vi "PS2000.vi"() -> ()   [LabVIEW 2016]
uses:
  <vilib>/measure/mascope.llb/Amplitude and Levels 1 chan.vi
  <vilib>/measure/matone.llb/Extract Single Tone Information 1 Chan.vi
  <vilib>/measure/mascope.llb/Pulse Measurements 1 chan.vi
  PS2000.dll
  <vilib>/measure/NI_MAPro.lvlib
panel:
  out "Phase":dbl
  out "Low level":dbl
  out "High level":dbl
  out "Amplitude":dbl
  out "Phase":dbl
  out "Behind":bool
  out "Advance":bool
  out "Low level":dbl
  out "High level":dbl
  out "Amplitude":dbl
  out "Phase difference":dbl
  out "Duty cycle":dbl
  out "Period":dbl
  out "Duty cycle":dbl
  out "Period":dbl
  in  "Voltage Range":dbl(knob) min=0.0 max=20.0 step=0.001 scale=0.0..20.0
  in  "Time":dbl(knob) min=0.0 max=1.0 step=0.0001 scale=0.0..1.0
  in  "stop 2":bool
  in  "Sweeps":u32
  in  "Sweep Type":u16(ring) items=["Up", "Down", "Up/Down", "Down/Up"]
  in  "Dwell Time":sgl
  in  "Increment":sgl
  in  "Stop Frequency":sgl=1000.0
  in  "Start Frequency":sgl=1000.0
  in  "Waveform Type":u16(ring) items=["Sine", "Square", "Triangle", "Rampup", "Rampdown"]
  in  "Peak to Peak":u32=1000000
  in  "Offset Voltage":i32
  in  "Source":i16(ring)=5 items=["Ch A", "Ch B", "Ch C", "Ch D", "Ext", "None"]
  in  "Voltage mV":i16=1400 min=0 max=20000 step=1
  out "Handle":u16
  out "Max number of samples you can use":i32=15871
  in  "Range":i16(ring)=5 items=["20V"=10, "10V"=9, "5V"=8, "2V"=7, "1V"=6, "500mV"=5, "200mV"=4, "100mV"=3, "50mV"=2]
  in  "Range":i16(ring)=8 items=["20V"=10, "10V"=9, "5V"=8, "2V"=7, "1V"=6, "500mV"=5, "200mV"=4, "100mV"=3, "50mV"=2]
  out "?":waveform(dbl)[](graph)=[{"t0"=timestamp(3286802554.3350306 s since 1904-01-01), "dt"=5.024e-05, "Y"=array[1256 elements]}, {"t0"=timestamp(3286802554.3350306 s since 1904-01-01), "dt"=5.024e-05, "Y"=array[1256 elements]}, {"t0"=timestamp(3286802554.3350306 s since 1904-01-01), "dt"=5.024e-05, "Y"=array[1256 elements]}, {"t0"=timestamp(3286802554.3350306 s since 1904-01-01), "dt"=5.024e-05, "Y"=array[1256 elements]}]
  in  "Enabled":bool
  in  "Enabled":bool=TRUE
  in  "DC":i16(ring) items=["AC", "DC"]
  in  "DC":i16(ring)=1 items=["AC", "DC"]
  in  "No. of samples":i32=1256 min=0
  in  "Timebase":i16=3 min=0 max=14 step=1
  in  "Auto Trigger ms":i16 min=0 max=5000 step=100
  in  "Delay":i16 min=-100 max=100 step=1
  in  "Direction":i16(ring) items=["Rising", "Falling"]
  in  "stop":bool
  # "Computer Oscilloscope"
  # "(Edition: Automatic Performance Test For Encoders )"
  # "Channel A"
  # "Channel B"
  # "Timebase"
  # "Trigger"
  # "AWG"
  # "Channel A"
  # "Channel B"
  # "Special function"
  # "V.2016.9.13.1"
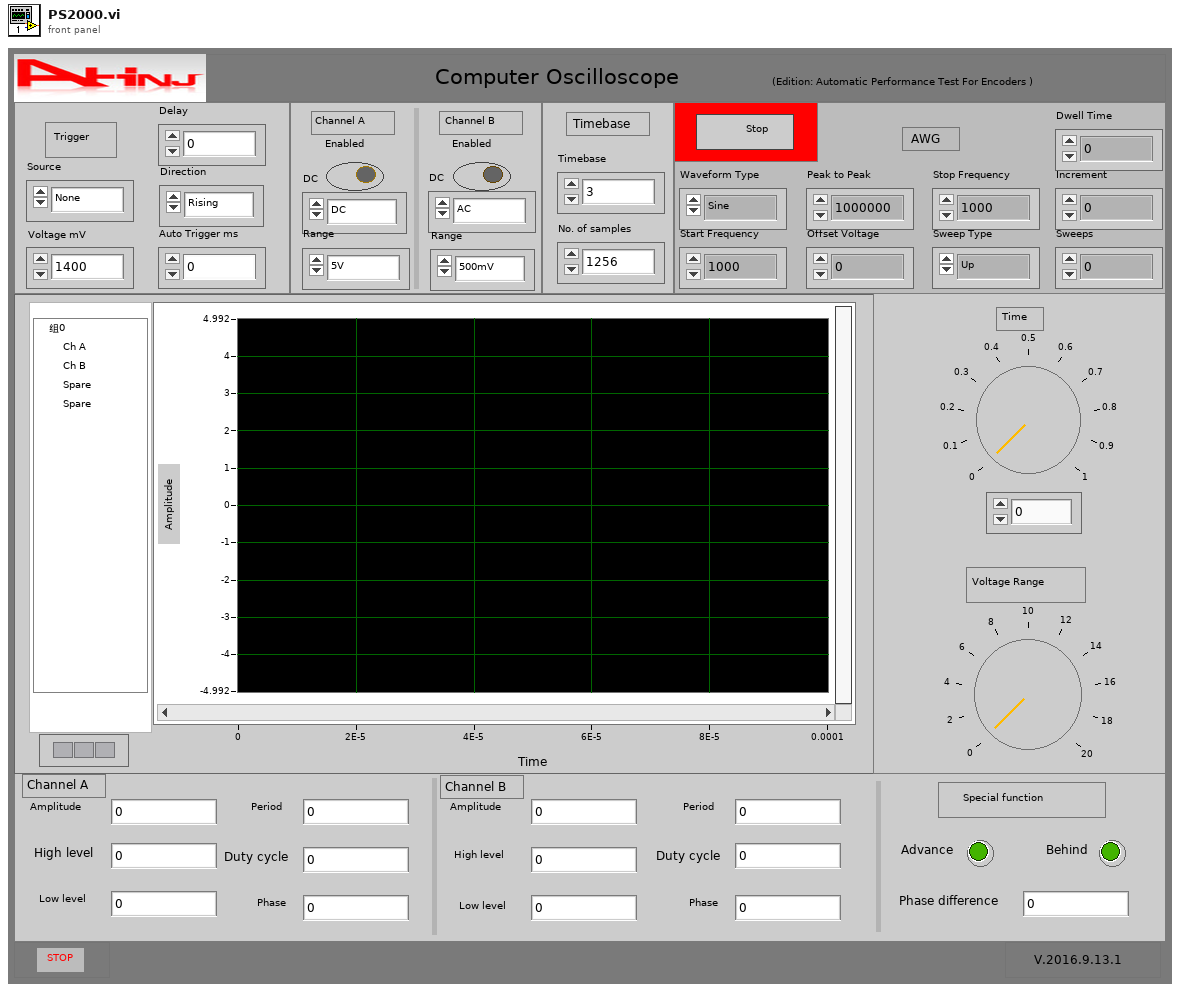
[diagram p1: front panel]
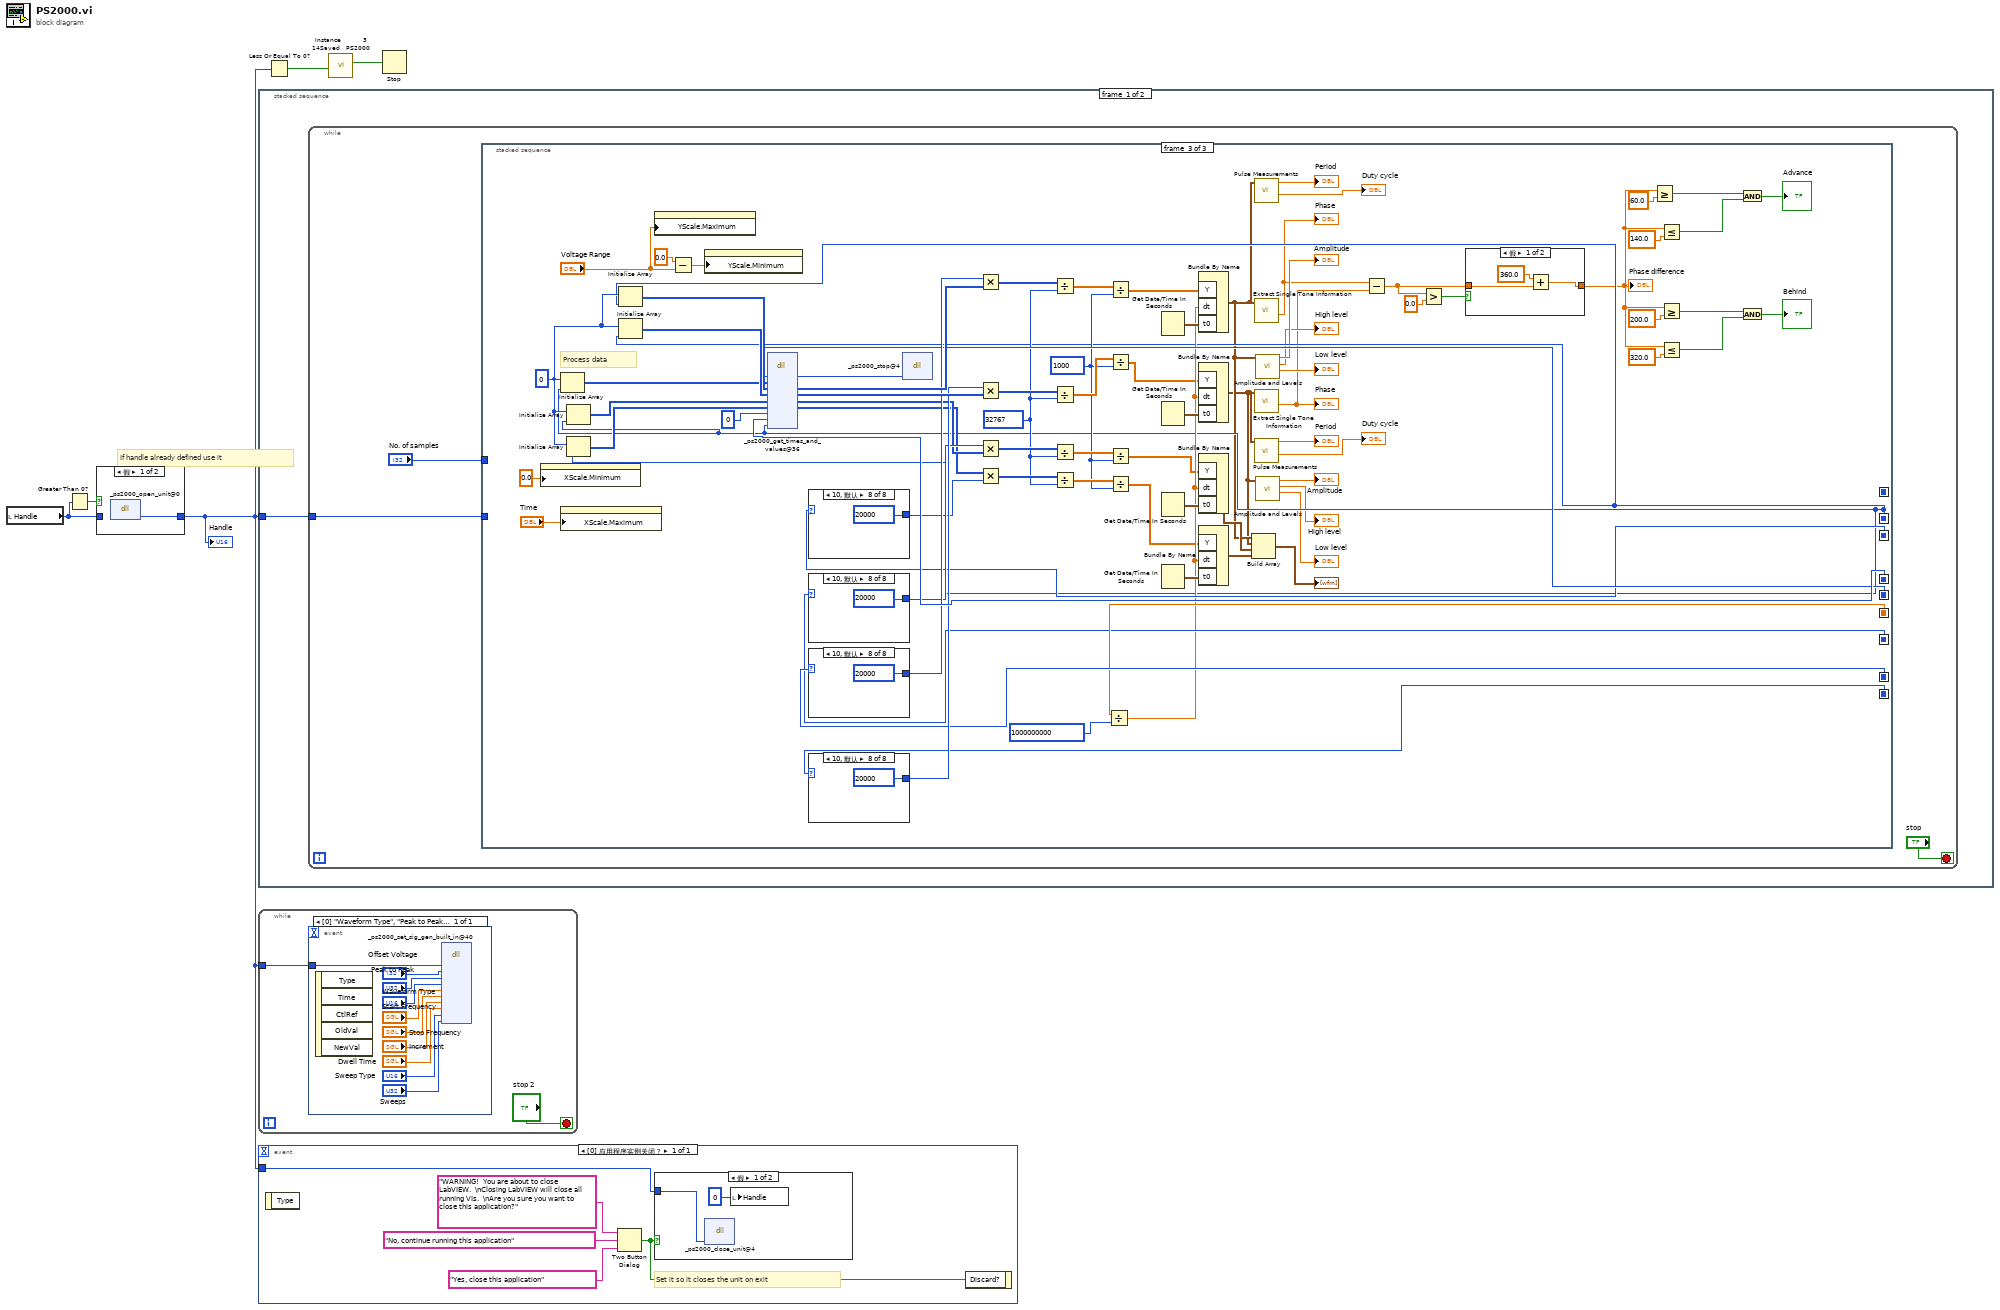
[diagram p0: block diagram]
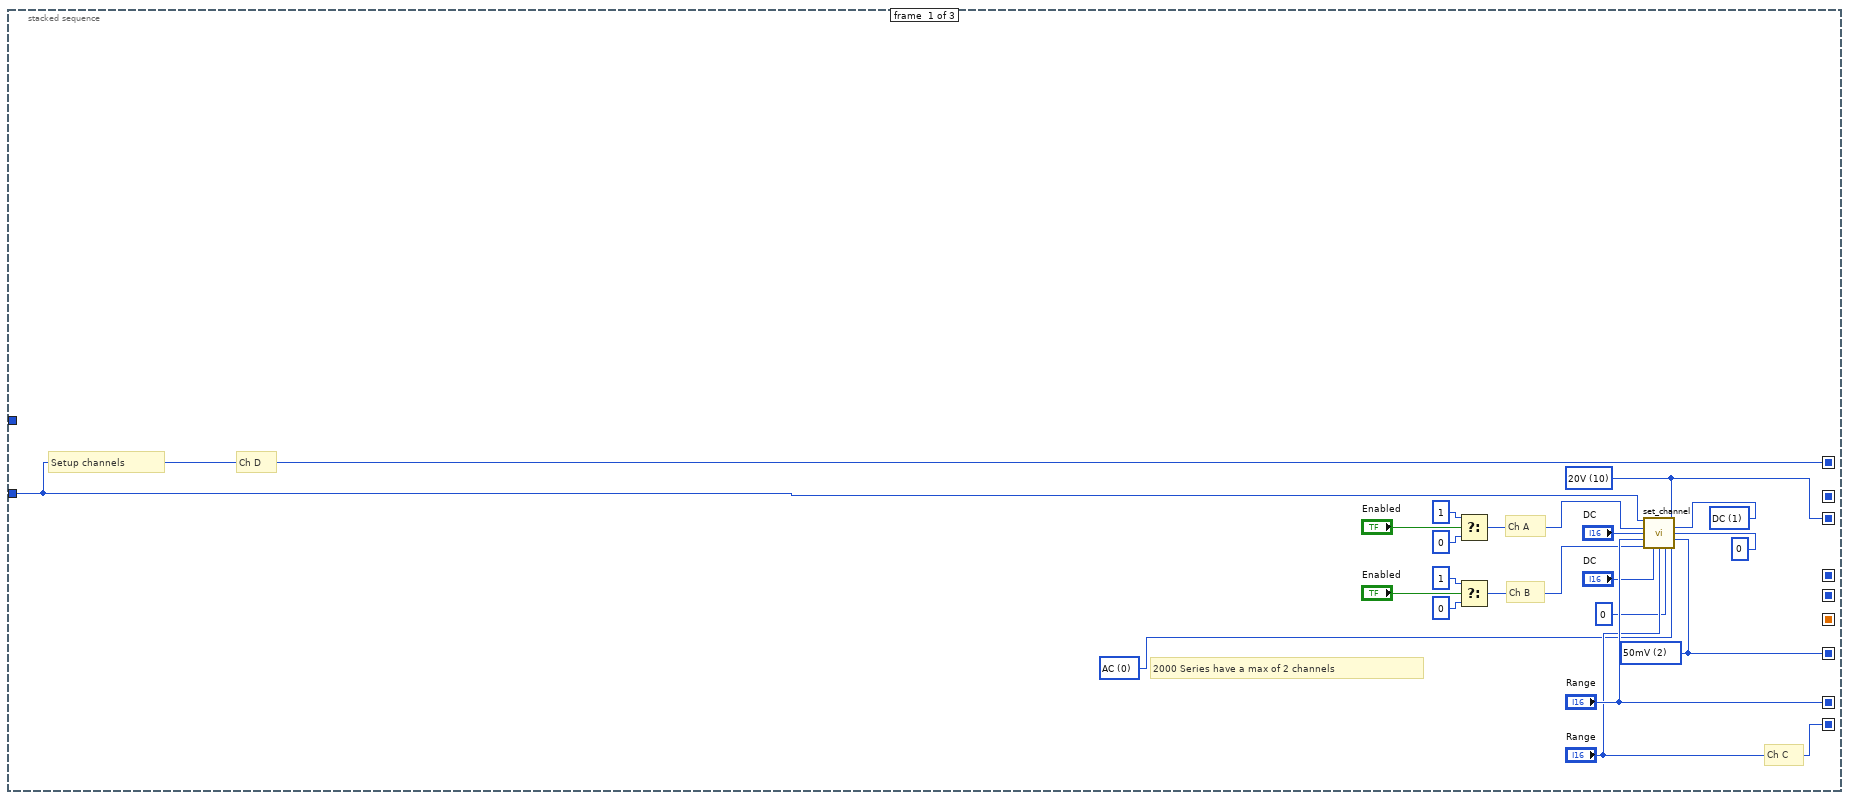
[diagram p3: hidden frame]
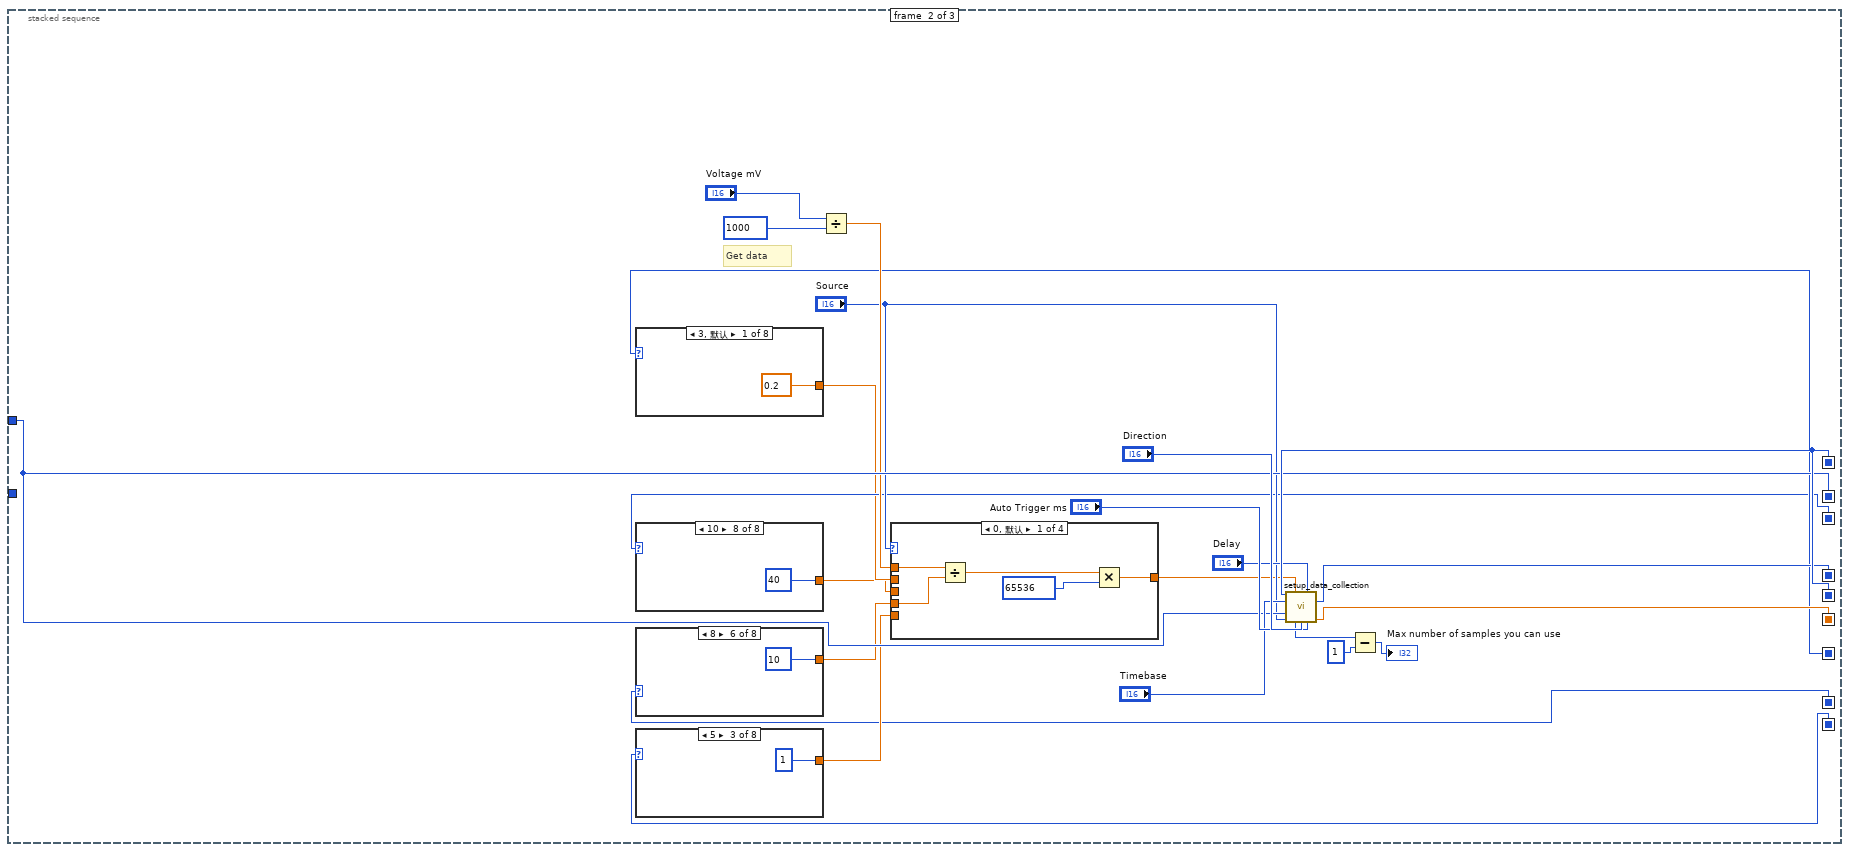
[diagram p4: hidden frame]
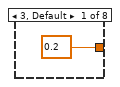
[diagram p5: hidden frame]
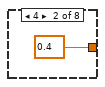
[diagram p6: hidden frame]
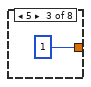
[diagram p7: hidden frame]
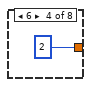
[diagram p8: hidden frame]
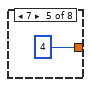
[diagram p9: hidden frame]
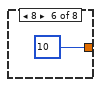
[diagram p10: hidden frame]
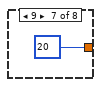
[diagram p11: hidden frame]
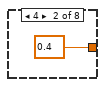
[diagram p12: hidden frame]
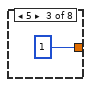
[diagram p13: hidden frame]
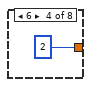
[diagram p14: hidden frame]
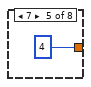
[diagram p15: hidden frame]
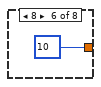
[diagram p16: hidden frame]
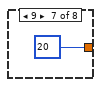
[diagram p17: hidden frame]
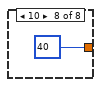
[diagram p18: hidden frame]
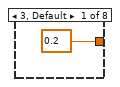
[diagram p19: hidden frame]
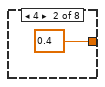
[diagram p20: hidden frame]
diagram:
  # "If handle already defined use it"
  n1 = local read "Handle"() -> (w4:u16)
  n2 = Greater Than 0?(x=w4) -> (x > 0?=w5:bool)
  n3 = case shown="假" w5 {
    tunnel: [w6 w7] -> w1
    tunnel: w4 -> [_ w7]
    frame False {
      n4 = dll-call lib="PS2000.dll" fn="_ps2000_open_unit@0" label="OpenUnit"() -> ("Handle"=w6:i16)  [unwired: 3 in, 2 out]
    }
    frame True {
    }
  }
  "Handle" <- w1
  n5 = stacked-sequence {
    tunnel: w1 -> [w8 _]
    frame #0 {
      n6 = while {
        tunnel: w8 -> [w10]
        stop <- "stop" stop-if-true
        n7 = stacked-sequence {
          seq-local: [w24 _ _] -> [_ w51 _]
          seq-local: [_ w51 _] -> [_ _ w168]
          seq-local: [_ w49 _] -> [_ _ w144]
          seq-local: [_ w50 _] -> [_ _ w182]
          seq-local: ["Range" _ _] -> [_ w36 w169]
          seq-local: ["Range" _ _] -> [_ w37 w170]
          seq-local: [_ w48 _] -> [_ _ w166]
          seq-local: [w15 _ _] -> [_ w34 w155]
          seq-local: [w14 _ _] -> [_ w33 w154]
          tunnel: w10 -> [w24 _ _]
          tunnel: "No. of samples" -> [_ w49 _]
          frame #0 {
            w16 = i16 1 items=["AC", "DC"] ("DC")
            w14 = i16 10 items=["20V"=10, "10V"=9, "5V"=8, "2V"=7, "1V"=6, "500mV"=5, "200mV"=4, "100mV"=3, "50mV"=2] ("Range")
            w17 = i16 0 items=["AC", "DC"] ("DC")
            w15 = i16 2 items=["20V"=10, "10V"=9, "5V"=8, "2V"=7, "1V"=6, "500mV"=5, "200mV"=4, "100mV"=3, "50mV"=2] ("Range")
            # "2000 Series have a max of 2 channels"
            # "Ch C"
            # "Ch D"
            # "Ch B"
            # "Ch A"
            # "Setup channels"
            n8 = Select(t=1, s="Enabled", f=0) -> (s? t:f=w23:i32)
            n9 = Select(t=1, s="Enabled", f=0) -> (s? t:f=w20:i32)
            n10 = call "set_channel.vi"("Handle"=w24, "Channel D range"=w14, "Channel A enabled"=w23, "Channel D dc"=w16, "Channel A dc"="DC", "Channel D enabled"=0, "Channel A range"="Range", "Channel C range"=w15, "Channel B enabled"=w20, "Channel B dc"="DC", "Channel B range"="Range", "Channel C enabled"=0, "Channel C dc"=w17) -> ()  [unwired: 3 in]
          }
          frame #1 {
            # "Get data"
            n11 = case shown="3, 默认" w34 {
              tunnel: [0.2 0.4 1 2 4 10 20 40] -> w32
              frame 3, Default {
              }
              frame 4 {
              }
              frame 5 {
              }
              frame 6 {
              }
              frame 7 {
              }
              frame 8 {
              }
              frame 9 {
              }
              frame 10 {
              }
            }
            n12 = case shown="10" w33 {
              tunnel: [0.2 0.4 1 2 4 10 20 40] -> w31
              frame 3, Default {
              }
              frame 4 {
              }
              frame 5 {
              }
              frame 6 {
              }
              frame 7 {
              }
              frame 8 {
              }
              frame 9 {
              }
              frame 10 {
              }
            }
            n13 = case shown="8" w36 {
              tunnel: [0.2 0.4 1 2 4 10 20 40] -> w40
              frame 3, Default {
              }
              frame 4 {
              }
              frame 5 {
              }
              frame 6 {
              }
              frame 7 {
              }
              frame 8 {
              }
              frame 9 {
              }
              frame 10 {
              }
            }
            n14 = case shown="5" w37 {
              tunnel: [0.2 0.4 1 2 4 10 20 40] -> w39
              frame 3, Default {
              }
              frame 4 {
              }
              frame 5 {
              }
              frame 6 {
              }
              frame 7 {
              }
              frame 8 {
              }
              frame 9 {
              }
              frame 10 {
              }
            }
            n15 = Divide(x="Voltage mV", y=1000) -> (x/y=w41:dbl)
            n16 = case shown="0, 默认" "Source" {
              tunnel: w40 -> [w90 _ _ _]
              tunnel: w39 -> [_ w92 _ _]
              tunnel: w41 -> [w91 w93 w98 w103]
              tunnel: [w87 w94 w99 w104] -> w35
              tunnel: w32 -> [_ _ w97 _]
              tunnel: w31 -> [_ _ _ w102]
              frame 0, Default {
                n17 = Divide(x=w91, y=w90) -> (x/y=w89:dbl)
                n18 = Multiply(x=w89, y=65536) -> (x*y=w87:dbl)
              }
              frame 1 {
                n19 = Divide(x=w93, y=w92) -> (x/y=w96:dbl)
                n20 = Multiply(x=w96, y=65536) -> (x*y=w94:dbl)
              }
              frame 2 {
                n21 = Divide(x=w98, y=w97) -> (x/y=w101:dbl)
                n22 = Multiply(x=w101, y=65536) -> (x*y=w99:dbl)
              }
              frame 3 {
                n23 = Divide(x=w103, y=w102) -> (x/y=w106:dbl)
                n24 = Multiply(x=w106, y=65536) -> (x*y=w104:dbl)
              }
            }
            n25 = call "setup_data_collection.vi"("Handle"=w51, "Threshold"=w35, "Delay"="Delay", "Timebase"="Timebase", "No of samples"=w49, "Source"="Source", "Direction"="Direction", "Auto Trigger ms"="Auto Trigger ms") -> ("time units"=w50:i16, "Max Samples"=w45:i32, "time_interval_ns"=w48:dbl)  [unwired: 3 in, 2 out]
            n26 = Subtract(x=w45, y=1) -> (x-y=→"Max number of samples you can use":i32)
          }
          frame #2 {
            w158 = 1000
            w159 = 32767
            w145 = 0
            # "Process data"
            n27 = property class="MixedGraph (严格)"("XScale.Minimum"=0.0) -> ()  [unwired: 2 in, 2 out]
            n28 = Initialize Array(w145, w144) -> (w142:i32[])
            n29 = property class="MixedGraph (严格)"("XScale.Maximum"="Time") -> ()  [unwired: 2 in, 2 out]
            n30 = Initialize Array(w145, w144) -> (w184:i32[])
            n31 = Initialize Array(w145, w144) -> (w183:i32[])
            n32 = Initialize Array(w145, w144) -> (w186:i32[])
            n33 = Initialize Array(w145, w144) -> (w185:i32[])
            n34 = property class="MixedGraph (严格)"("YScale.Maximum"="Voltage Range") -> ()  [unwired: 2 in, 2 out]
            n35 = Subtract(x=0.0, y="Voltage Range") -> (x-y=w139:dbl)
            n36 = property class="MixedGraph (严格)"("YScale.Minimum"=w139) -> ()  [unwired: 2 in, 2 out]
            n37 = dll-call lib="PS2000.dll" fn="_ps2000_get_times_and_values@36" label="GetTimes&Values"("handle"=w168, "times"=w142, "bufferA"=w186, "bufferB"=w185, "bufferC"=w184, "bufferD"=w183, "overflow"=0, "times_units"=w182, "numValues"=w144) -> ("handle"=w178:i16, "bufferA"=w179:i16[], "bufferB"=w173:i16[], "bufferC"=w157:i16[], "bufferD"=w156:i16[])  [unwired: 8 in, 2 out]
            n38 = case shown="10, 默认" w154 {
              tunnel: [100 200 500 1000 2000 5000 10000 20000] -> w160
              frame 3 {
              }
              frame 4 {
              }
              frame 5 {
              }
              frame 6 {
              }
              frame 7 {
              }
              frame 8 {
              }
              frame 9 {
              }
              frame 10, Default {
              }
            }
            n39 = case shown="10, 默认" w155 {
              tunnel: [100 200 500 1000 2000 5000 10000 20000] -> w161
              frame 3 {
              }
              frame 4 {
              }
              frame 5 {
              }
              frame 6 {
              }
              frame 7 {
              }
              frame 8 {
              }
              frame 9 {
              }
              frame 10, Default {
              }
            }
            n40 = case shown="10, 默认" w169 {
              tunnel: [100 200 500 1000 2000 5000 10000 20000] -> w171
              frame 3 {
              }
              frame 4 {
              }
              frame 5 {
              }
              frame 6 {
              }
              frame 7 {
              }
              frame 8 {
              }
              frame 9 {
              }
              frame 10, Default {
              }
            }
            n41 = case shown="10, 默认" w170 {
              tunnel: [100 200 500 1000 2000 5000 10000 20000] -> w172
              frame 3 {
              }
              frame 4 {
              }
              frame 5 {
              }
              frame 6 {
              }
              frame 7 {
              }
              frame 8 {
              }
              frame 9 {
              }
              frame 10, Default {
              }
            }
            n42 = dll-call lib="PS2000.dll" fn="_ps2000_stop@4" label="Stop"("handle"=w178) -> ()  [unwired: 5 in, 2 out]
            n43 = Multiply(x=w171, y=w179) -> (x*y=w181:i32[])
            n44 = Multiply(x=w172, y=w173) -> (x*y=w176:i32[])
            n45 = Multiply(x=w161, y=w157) -> (x*y=w165:i32[])
            n46 = Multiply(x=w156, y=w160) -> (x*y=w163:i32[])
            n47 = Divide(x=w181, y=w159) -> (x/y=w180:dbl[])
            n48 = Divide(x=w176, y=w159) -> (x/y=w175:dbl[])
            n49 = Divide(x=w165, y=w159) -> (x/y=w164:dbl[])
            n50 = Divide(x=w163, y=w159) -> (x/y=w162:dbl[])
            n51 = Divide(x=w166, y=1000000000) -> (x/y=w151:dbl)
            n52 = Divide(x=w180, y=w158) -> (x/y=w125:dbl[])
            n53 = Divide(x=w175, y=w158) -> (x/y=w136:dbl[])
            n54 = Divide(x=w164, y=w158) -> (x/y=w147:dbl[])
            n55 = Divide(x=w162, y=w158) -> (x/y=w146:dbl[])
            n56 = Get Date/Time In Seconds() -> (seconds since 1Jan1904=w177:timestamp)
            n57 = Get Date/Time In Seconds() -> (seconds since 1Jan1904=w174:timestamp)
            n58 = Get Date/Time In Seconds() -> (seconds since 1Jan1904=w153:timestamp)
            n59 = Get Date/Time In Seconds() -> (seconds since 1Jan1904=w152:timestamp)
            n60 = Bundle By Name("Y"=w125, "dt"=w151, "t0"=w177) -> (w113:waveform(dbl))  [unwired: 1 in]
            n61 = Bundle By Name("Y"=w136, "dt"=w151, "t0"=w174) -> (w111:waveform(dbl))  [unwired: 1 in]
            n62 = Bundle By Name("Y"=w147, "dt"=w151, "t0"=w153) -> (w149:waveform(dbl))  [unwired: 1 in]
            n63 = Bundle By Name("Y"=w146, "dt"=w151, "t0"=w152) -> (w150:waveform(dbl))  [unwired: 1 in]
            n64 = Build Array(w113, w111, w149, w150) -> (→"?":waveform(dbl)[])
            n65 = call-poly <vilib>:"Pulse Measurements.vi"("signal in"=w113) -> ("duty cycle"=→"Duty cycle":dbl, "period"=→"Period":dbl)  [unwired: 6 in, 3 out]
            n66 = call-poly <vilib>:"Extract Single Tone Information.vi"("time signal in"=w113) -> ("detected phase (deg)"=w112:dbl)  [unwired: 5 in, 5 out]
            "Phase" <- w112
            n67 = call-poly <vilib>:"Extract Single Tone Information.vi"("time signal in"=w111) -> ("detected phase (deg)"=w107:dbl)  [unwired: 5 in, 5 out]
            "Phase" <- w107
            n68 = call-poly <vilib>:"Pulse Measurements.vi"("signal in"=w111) -> ("duty cycle"=→"Duty cycle":dbl, "period"=→"Period":dbl)  [unwired: 6 in, 3 out]
            n69 = call-poly <vilib>:"Amplitude and Levels.vi"("signal in"=w113) -> ("low state level"=→"Low level":dbl, "high state level"=→"High level":dbl, "amplitude"=→"Amplitude":dbl)  [unwired: 7 in, 1 out]
            n70 = call-poly <vilib>:"Amplitude and Levels.vi"("signal in"=w111) -> ("low state level"=→"Low level":dbl, "high state level"=→"High level":dbl, "amplitude"=→"Amplitude":dbl)  [unwired: 7 in, 1 out]
            n71 = Subtract(x=w112, y=w107) -> (x-y=w129:dbl)
            n72 = Greater?(x=w129, y=0.0) -> (0:w130:bool)
            n73 = case shown="假" w130 {
              tunnel: w129 -> [w189 w190]
              tunnel: [w187 w190] -> w116
              frame False {
                n74 = Add(x=360.0, y=w189) -> (x+y=w187:dbl)
              }
              frame True {
              }
            }
            "Phase difference" <- w116
            n75 = Greater Or Equal?(x=w116, y=60.0) -> (x >= y?=w121:bool)
            n76 = Less Or Equal?(x=w116, y=140.0) -> (x <= y?=w122:bool)
            n77 = Greater Or Equal?(x=w116, y=200.0) -> (x >= y?=w118:bool)
            n78 = Less Or Equal?(x=w116, y=320.0) -> (x <= y?=w119:bool)
            n79 = And(x=w121, y=w122) -> (x .and. y?=→"Advance":bool)
            n80 = And(x=w118, y=w119) -> (x .and. y?=→"Behind":bool)
          }
        }
      }
    }
    frame #1 {
      n81 = Stop(stop? (T)=TRUE) -> ()
    }
  }
  n82 = while {
    tunnel: w1 -> [w225]
    stop <- "stop 2" stop-if-true
    n83 = event shown="[0] \"Waveform Type\", \"Peak to Peak\", \"Offset Voltage\", \"Stop Frequency\", \"Increment\", \"Dwell Time\", \"Sweep Type\", \"Sweeps\": 值改变" {
      selector: _ -> [_]
      dyn-events: _ -> [_]
      timeout: _ -> [_]
      tunnel: w225 -> [w226]
      event "Waveform Type", "Peak to Peak", "Offset Voltage", "Stop Frequency", "Increment", "Dwell Time", "Sweep Type", "Sweeps": Value Change {
        n84 = event-data() -> ()  [unwired: 1 in, 5 out]
        n85 = dll-call lib="PS2000.dll" fn="_ps2000_set_sig_gen_built_in@40"("handle"=w226, "offsetvoltage"="Offset Voltage", "pktopk"="Peak to Peak", "wavetype"="Waveform Type", "startfrequency"="Start Frequency", "stopfrequency"="Stop Frequency", "increment"="Increment", "dwelltime"="Dwell Time", "sweeptype"="Sweep Type", "sweeps"="Sweeps") -> ()  [unwired: 14 in, 2 out]
      }
    }
  }
  n86 = event shown="[0] 应用程序实例关闭？" {
    selector: _ -> [_]
    dyn-events: _ -> [_]
    timeout: _ -> [_]
    tunnel: w1 -> [w236]
    event Application Instance Close? {
      # "Set it so it closes the unit on exit"
      n87 = event-data() -> ()  [unwired: 1 in, 1 out]
      n88 = Two Button Dialog(message="WARNING!  You are about to close LabVIEW.  \nClosing LabVIEW will close all running VIs.  \nAre you sure you want to close this application?", 1:"Yes, close this application" ("F button name (\"Cancel\")"), 2:"No, continue running this application" ("T button name (\"OK\")")) -> (T button?=w237:bool)
      n89 = case shown="假" w237 {
        tunnel: w236 -> [w241 _]
        frame False {
          n90 = dll-call lib="PS2000.dll" fn="_ps2000_close_unit@4" ("ps3000.dll:_ps3000_close_unit@4")("handle"=w241) -> ()  [unwired: 5 in, 2 out]
          n91 = local write "Handle"(0) -> ()
        }
        frame True {
        }
      }
      n92 = event-data("Discard?"=w237) -> ()  [unwired: 1 in, 1 out]
    }
  }
  n93 = Less Or Equal To 0?(x=w1) -> (x <= 0?=w2:bool)
  n94 = call "Instance           3 14Saved   PS2000 .vi"("Enable"=w2) -> ("OK"=w3:bool)  [unwired: 9 in, 1 out]
  n95 = Stop(stop? (T)=w3) -> ()
